vi "AdvancedConfig.vi"(8 "error in":errorcluster {"code" format="Error %.0f"}, 11 "MainFGV_data":T2) -> (0 "error out":errorcluster {"code" format="Error %.0f"}, 3 "MainFGV_data out":T2)   [LabVIEW 2016]
uses:
  MainFGV_data.ctl
  config_board.ctl
panel:
  in  "Filtro":T1(ring)
  in  "cutoff":dbl=-3.0 caption="Cutoff amplitude [dB]"
  in  "preTrigger":dbl=0.1 caption="Pre-trigger [s]"
  in  "thr":dbl=100.0 caption="Limiar de força [N]"
  in  "integrationTime":dbl=1.0 caption="Tempo de integração [s]"
  in  "cancel":bool
  in  "ok":bool
  in  "rate":dbl=1000.0 caption="Taxa de aquisição [Hz]"
  # "Configurações avançadas"
  # "Apresentação do resultado"
  # "Detecção da batida"
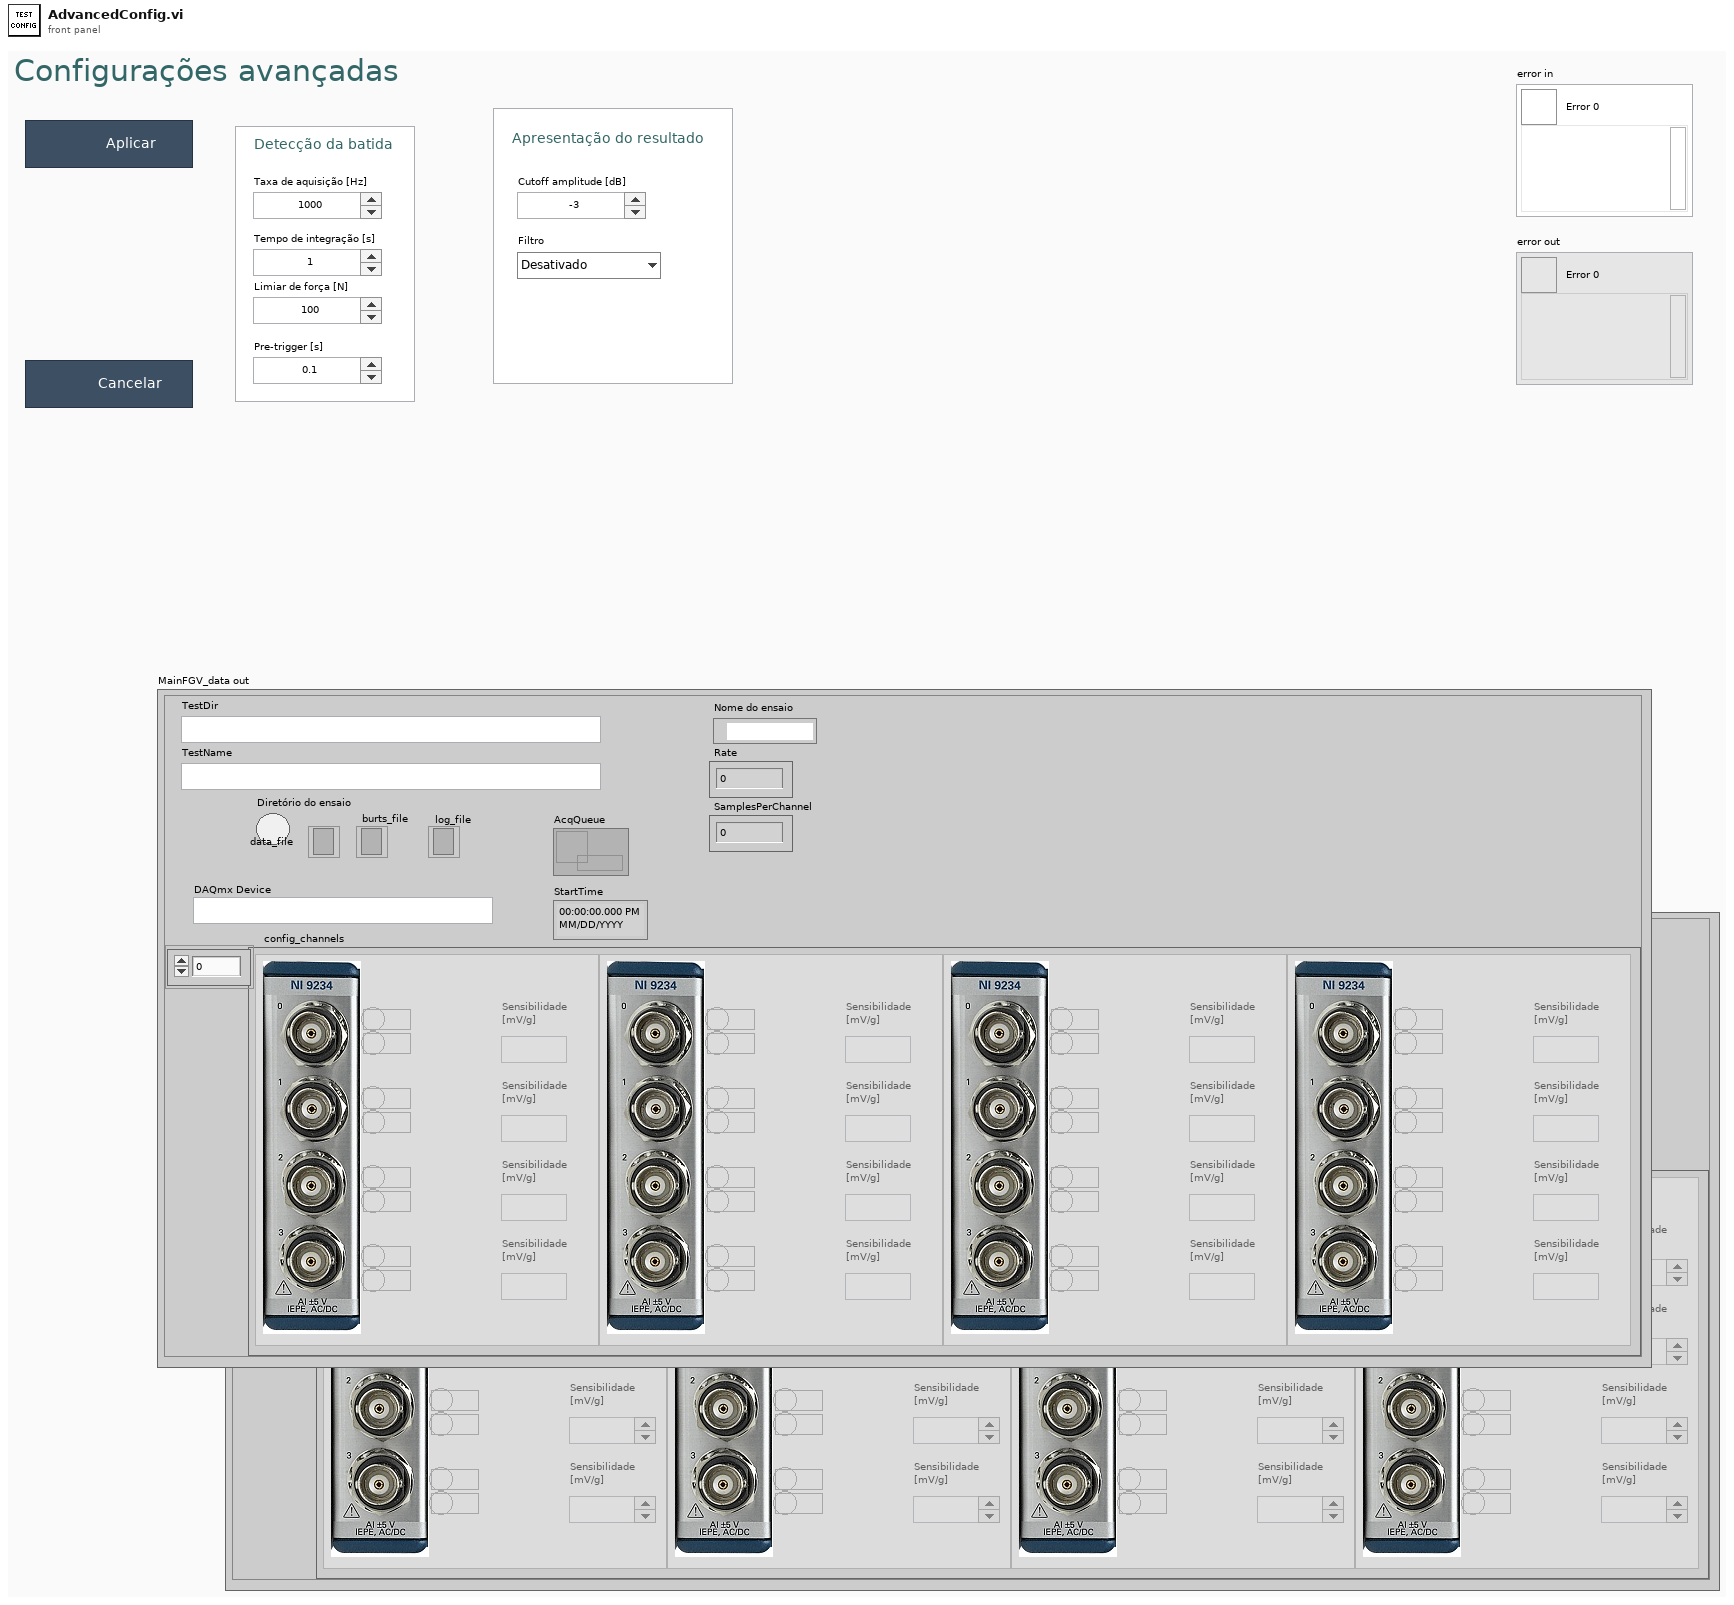
[diagram p1: front panel]
types:
  T1 = enum16{"Desativado", "Passa banda", "Passa alta", "Passa baixa"}
  T2 = typedef "MainFGV_data.ctl" = cluster{"TestDir":path, "TestName":string, "Simulation":bool, "task":refnum<k21>, "data_file":refnum<file>, "burts_file":refnum<file>, "log_file":refnum<file>, "Rate":dbl, "SamplesPerChannel":dbl, "AcqQueue":refnum<queue>, "StartTime":timestamp, "config_channels":T3[], "DAQmx Device":tag}
  T3 = typedef "config_board.ctl" = cluster{"Sens 1":dbl, "active 1":bool, "type 1":bool, "type 2":bool, "active 2":bool, "Sens 2":dbl, "type 3":bool, "active 3":bool, "Sens 3":dbl, "type 4":bool, "active 4":bool, "Sens 4":dbl}
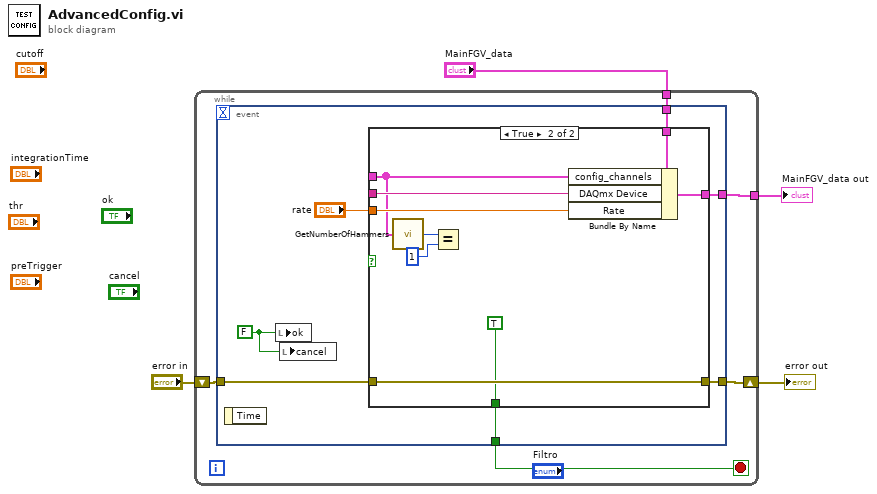
[diagram p0: block diagram]
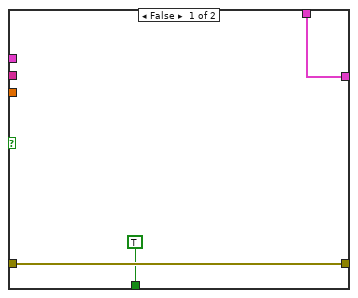
[diagram p2: hidden frame]
diagram:
  n1 = while {
    shift-right: [w7] -> w3
    shift-left: "error in" -> [w8]
    tunnel: "MainFGV_data" -> [w6]
    tunnel: [w5] -> w1
    stop <- w9 stop-if-true
    n2 = event {
      selector: _ -> [_]
      dyn-events: _ -> [_]
      timeout: _ -> [_]
      tunnel: [w10] -> w9
      tunnel: w8 -> [w15]
      tunnel: [w14] -> w7
      tunnel: w6 -> [w19]
      tunnel: [w18] -> w5
      event #0 {
        w17 = FALSE ("OK")
        n3 = event-data() -> ()  [unwired: 1 in, 1 out]
        n4 = local write "ok"(w17) -> ()
        n5 = local write "cancel"(w17) -> ()
        n6 = case shown="True" w16 {
          tunnel: [_ w31] -> w13
          tunnel: [_ w26] -> w11
          tunnel: w19 -> [w22 w30]
          tunnel: [w22 w29] -> w18
          tunnel: w15 -> [w21 w28]
          tunnel: [w21 w28] -> w14
          tunnel: "rate" -> [_ w27]
          tunnel: [TRUE ("OK") TRUE ("OK")] -> w10
          frame False {
          }
          frame True {
            n7 = call "GetNumberOfHammers.vi"("config"=w26) -> ("hammers"=w25:i16)  [unwired: 4 in]
            n8 = Equal?(x=w25, y=i16 1) -> ()  [unwired: 1 out]
            n9 = Bundle By Name(cluster=w30, "config_channels"=w26, "DAQmx Device"=w31, "Rate"=w27) -> (w29:T2)
          }
        }
      }
    }
  }
  "MainFGV_data out" <- w1
  "error out" <- w3
